vi "Write Signal Ref.vi"(8 "error in (no error)":errorcluster, 10 "Signal Ref":refnum<vi>, 11 "Abstract Saver in":refnum<class "Abstract Saver.lvclass">) -> (0 "error out":errorcluster, 3 "Abstract Saver out":refnum<class "Abstract Saver.lvclass">)   [LabVIEW 2016, in "Data Saving.lvlib" / "Abstract Saver.lvclass"]
uses:
  Abstract Saver.lvclass
  Abstract Saver.lvclass/Abstract Saver.ctl
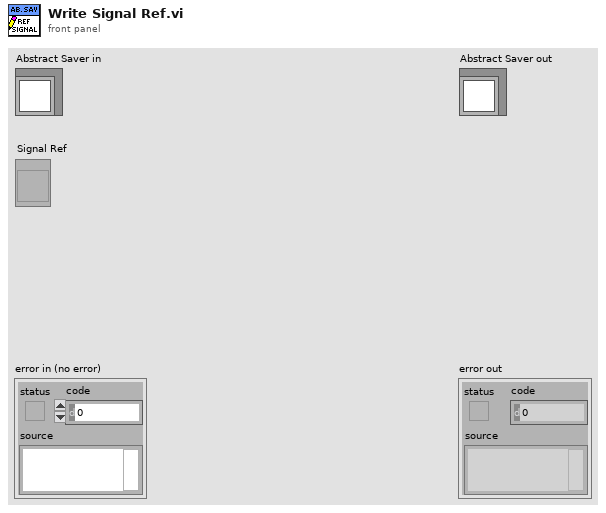
[diagram p1: front panel]
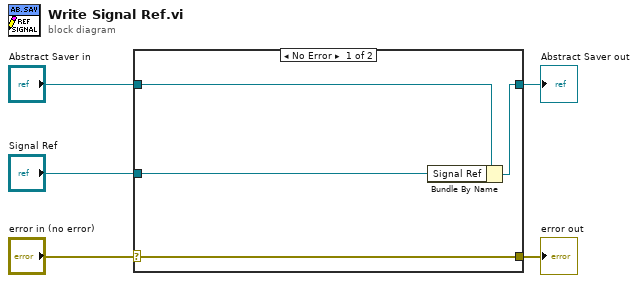
[diagram p0: block diagram]
diagram:
  n1 = case shown="No Error" "error in (no error)" {
    selector: "error in (no error)" -> [w9 w10]
    tunnel: [w9 w10] -> w4
    tunnel: [w7 w11] -> w2
    tunnel: "Abstract Saver in" -> [w8 w11]
    tunnel: "Signal Ref" -> [w6 _]
    frame No Error {
      n2 = Bundle By Name(cluster=w8, "Signal Ref"=w6) -> (w7:refnum<class "Abstract Saver.lvclass">)
    }
    frame Error {
    }
  }
  "error out" <- w4
  "Abstract Saver out" <- w2
